vi "Parse Basic Response.vi"(8 "error in (no error)":errorcluster, 11 "body in":string) -> (0 "error out":errorcluster, 2 "result cluster":T1, 3 "body out":string)   [LabVIEW 2014, in "Random JSON API.lvlib"]
uses:
  Random JSON API.lvlib
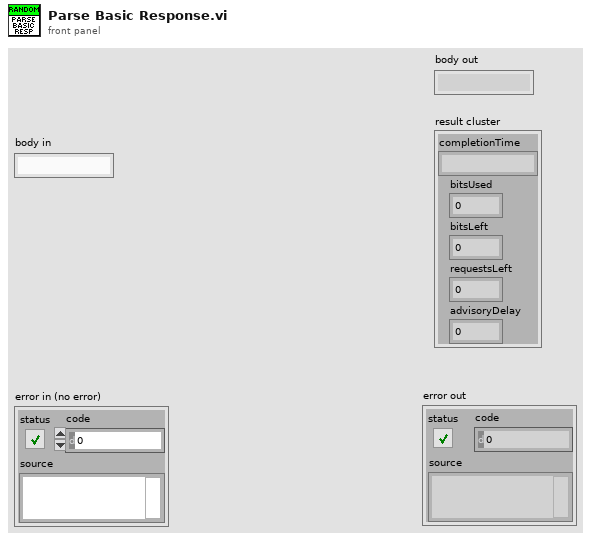
[diagram p1: front panel]
types:
  T1 = cluster{"completionTime":string, "bitsUsed":i32, "bitsLeft":i32, "requestsLeft":i32, "advisoryDelay":i32}
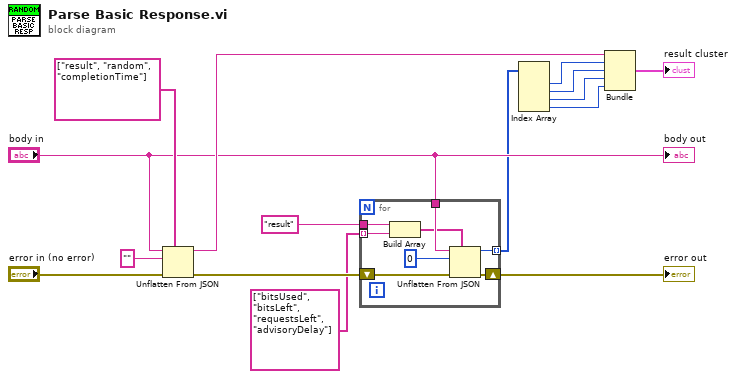
[diagram p0: block diagram]
diagram:
  n1 = Unflatten From JSON(path=string[] ["result", "random", "completionTime"], JSON string="body in", type and defaults="", error in (no error)="error in (no error)") -> (value=w11:string, error out=w10:errorcluster)  [unwired: 3 in]
  n2 = for {
    tunnel: "body in" -> [w21]
    shift-right: [w22] -> w9
    shift-left: w10 -> [w23]
    tunnel: [w19] -> w7 mode=indexing
    tunnel: "result" -> [w18]
    tunnel: string[] ["bitsUsed", "bitsLeft", "requestsLeft", "advisoryDelay"] -> [w16] mode=indexing
    n3 = Build Array(w18, w16) -> (w17:string[])
    n4 = Unflatten From JSON(path=w17, JSON string=w21, type and defaults=0, error in (no error)=w23) -> (value=w19:i32, error out=w22:errorcluster)  [unwired: 3 in]
  }
  "error out" <- w9
  n5 = Index Array(array=w7) -> (element #1=w6:i32, element #2=w5:i32, element #3=w4:i32, element #4=w3:i32)  [unwired: 4 in]
  n6 = Bundle(w11, w6, w5, w4, w3) -> (→"result cluster":cluster{string, i32, i32, i32, i32})  [unwired: 1 in]
  "body out" <- "body in"
